vi "FTW-SyncServer-Destroy.vi"(0 "FTW Synchronous Server":refnum<data-value>, 11 "error in":errorcluster) -> (15 "error out":errorcluster)   [LabVIEW 2015]
uses:
  core/FTW-SyncServer-Core-Type.ctl
panel:
  # "Inputs"
  # "Outputs"
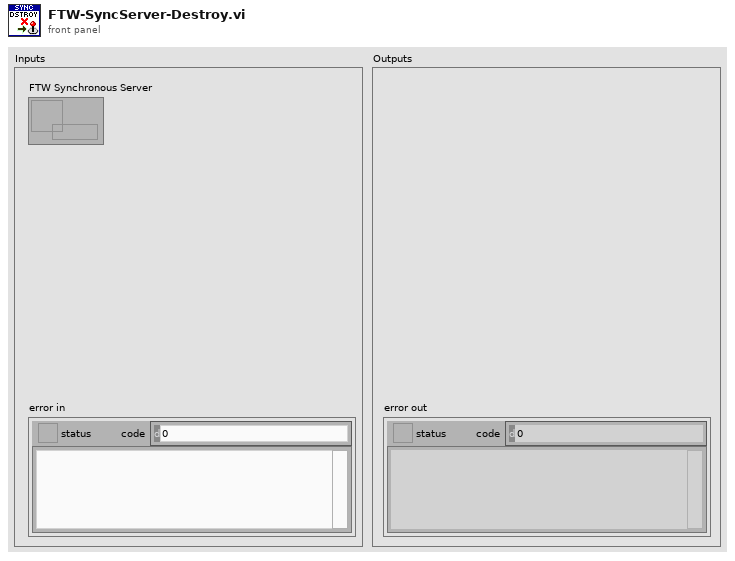
[diagram p1: front panel]
types:
  T1 = typedef "FTW-SyncServer-Core-Type.ctl" = cluster{"Socket":i64}
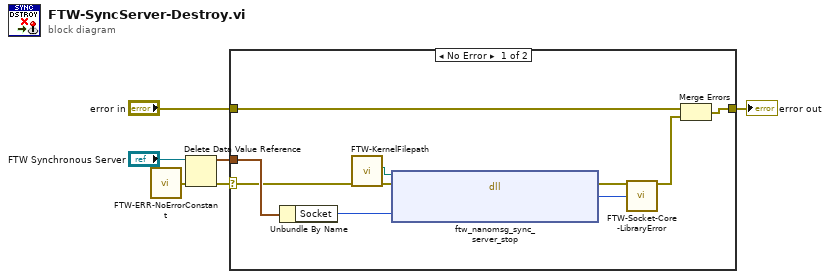
[diagram p0: block diagram]
diagram:
  n1 = call "FTW-ERR-NoErrorConstant.vi"() -> ("no error"=w1:errorcluster)
  n2 = Delete Data Value Reference(data value reference="FTW Synchronous Server", error in=w1) -> (data value=w3:T1, error out=w2:errorcluster)
  n3 = case shown="No Error" w2 {
    selector: w2 -> [w9 _]
    tunnel: [w16 w17] -> w6
    tunnel: "error in" -> [w14 w17]
    tunnel: w3 -> [w12 _]
    frame No Error {
      n4 = Unbundle By Name(w12) -> ("Socket"=w13:i64)
      n5 = call "FTW-KernelFilepath.vi"("error in"=w9) -> ("error out"=w8:errorcluster, "Library Filepath"=w7:path)  [unwired: 8 in, 1 out]
      n6 = dll-call lib="?" fn="ftw_nanomsg_sync_server_stop"(path in=w7, error in=w8, "Socket Handle"=w13) -> (error out=w11:errorcluster, "Return Value"=w10:i64)  [unwired: 2 in, 1 out]
      n7 = call "FTW-Socket-Core-LibraryError.vi"("error in"=w11, "Return Value"=w10) -> ("error out"=w15:errorcluster)  [unwired: 13 in]
      n8 = Merge Errors(w14, w15) -> (w16:errorcluster)
    }
    frame Error {
    }
  }
  "error out" <- w6
